vi "General_Slice 1D Array (U32).vi"(8 "Error":errorcluster, 9 "Slice":string caption="subset (i:j)", 11 "Array":u32[](array[colorbox])) -> (0 "Error Out":errorcluster, 3 "Array Out":u32[](array[colorbox]))   [LabVIEW 2009]
doc: "Modified OpenG vi Slice a 1D color array"
panel:
  # "Slice 1D Array.vi\n\nReturns a subset from array\n\nPlease visit http://www.OpenG.org to learn about the\nOpen Source LabVIEW software movement.\n\nNOTICE -- YOU MUST LEAVE THIS NOTICE IN PLACE.  PER THE TERMS OF THE LICENSE BELOW, YOU MAY SUBLICENSE THIS SOFTWARE \nIN ANY WAY THAT DOES NOT CONFLICT WITH THIS LICENSE.\n\n### BSD License (http://www.opensource.org/licenses/bsd-license.php) Begin ###\n \nCopyright (c) 2002, Jim Kring <jim@jimkring.com>\nCopyright (c) 2002, Cal-Bay Systems, Inc. <info@calbay.com>\n\nAll rights reserved.\n\nRedistribution and use in source and binary forms, with or without modification, are permitted provided that the following conditions are met:\n\n    * Redistributions of source code must retain the above copyright notice, this list of conditions and the following disclaimer.\n    * Redistributions in binary form must reproduce the above copyright notice, this list of conditions and the following disclaimer in the \n       documentation and/or other materials provided with the distribution.\n    * Neither the name of SciWare, James Kring, Inc., nor the names of its contributors may be used to endorse or promote products derived \n       from this software without specific prior written permission.\n\nTHIS SOFTWARE IS PROVIDED BY THE COPYRIGHT HOLDERS AND CONTRIBUTORS \"AS IS\" AND ANY EXPRESS OR IMPLIED WARRANTIES, \nINCLUDING, BUT NOT LIMITED TO, THE IMPLIED WARRANTIES OF MERCHANTABILITY AND FITNESS FOR A PARTICULAR PURPOSE ARE \nDISCLAIMED. IN NO EVENT SHALL THE COPYRIGHT OWNER OR CONTRIBUTORS BE LIABLE FOR ANY DIRECT, INDIRECT, INCIDENTAL,\n SPECIAL, EXEMPLARY, OR CONSEQUENTIAL DAMAGES (INCLUDING, BUT NOT LIMITED TO, PROCUREMENT OF SUBSTITUTE GOODS OR \nSERVICES; LOSS OF USE, DATA, OR PROFITS; OR BUSINESS INTERRUPTION) HOWEVER CAUSED AND ON ANY THEORY OF LIABILITY, \nWHETHER IN CONTRACT, STRICT LIABILITY, OR TORT (INCLUDING NEGLIGENCE OR OTHERWISE) ARISING IN ANY WAY OUT OF THE USE \nOF THIS SOFTWARE, EVEN IF ADVISED OF THE POSSIBILITY OF SUCH DAMAGE.\n\n### BSD License End ###"
  # "[OpenG VI Tags] ***Do Not Remove***\nSVN Revision = 593\nSVN Revision Date = 2007-01-18 16:52:28 -0800 (Thu, 18 Jan 2007)\nPackage = oglib_array-2.7-1\nDepends = oglib_string-2.6-1"
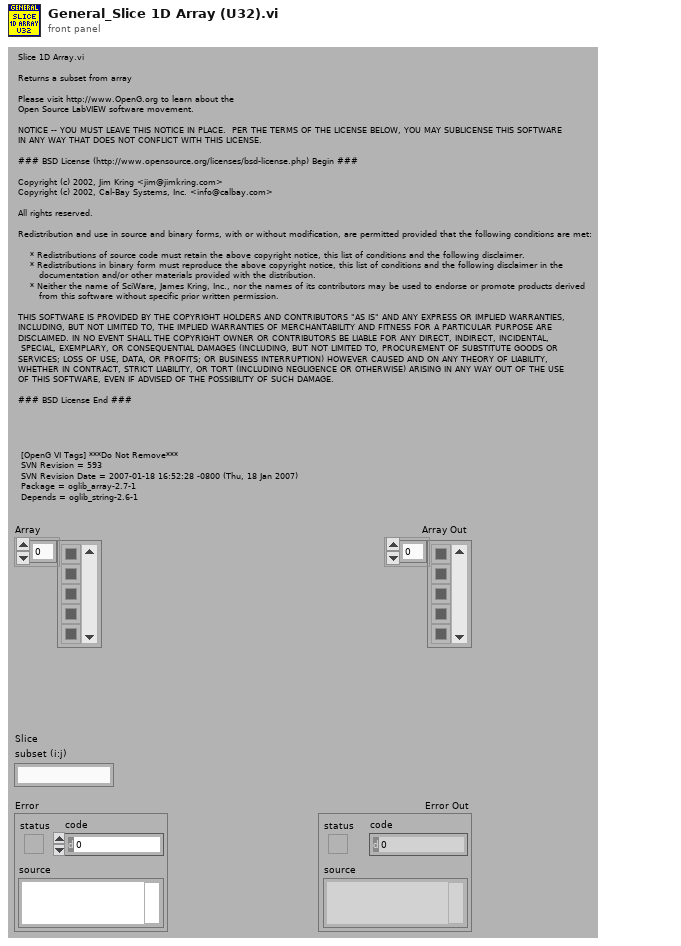
[diagram p1: front panel]
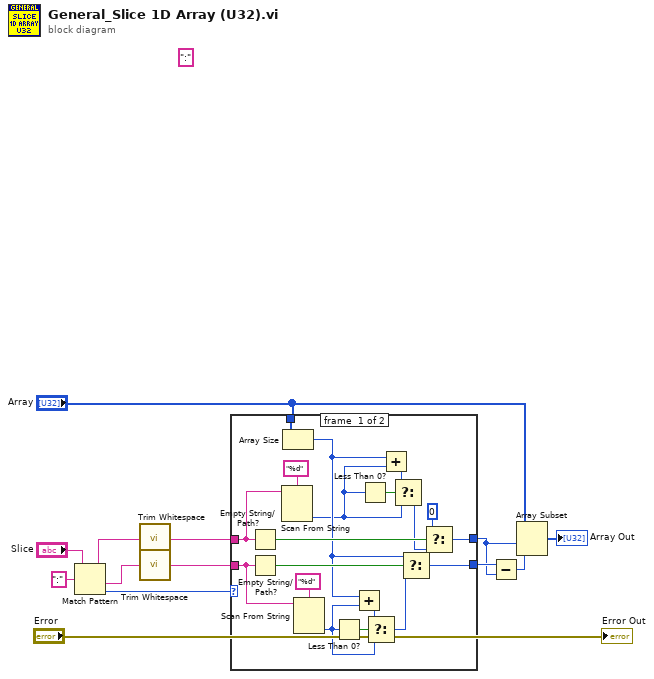
[diagram p0: block diagram]
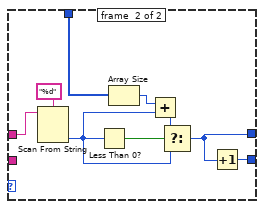
[diagram p2: hidden frame]
diagram:
  (unwired) ":"
  n1 = Match Pattern(string="Slice", regular expression=":" ("search string/char (-)")) -> (before substring=w7:string, after substring=w5:string, offset past match=w8:i32)  [unwired: 1 in, 1 out]
  n2 = call <vilib>:"Trim Whitespace.vi"("string"=w7) -> ("trimmed string"=w6:string)  [unwired: 1 in]
  n3 = call <vilib>:"Trim Whitespace.vi"("string"=w5) -> ("trimmed string"=w4:string)  [unwired: 1 in]
  n4 = case shown="-1" w8 {
    tunnel: [w23 w34] -> w13
    tunnel: [w24 w33] -> w12
    tunnel: "Array" -> [w29 w39]
    tunnel: w6 -> [w26 w40]
    tunnel: w4 -> [w30 _]
    frame #0 {
      n5 = Empty String/Path?(string/path=w26) -> (empty?=w28:bool)
      n6 = Empty String/Path?(string/path=w30) -> (empty?=w32:bool)
      n7 = Scan From String(format string="%d" ("Format String"), input string=w26) -> (output 1=w15:i32)  [unwired: 3 in, 3 out]
      n8 = Array Size(array=w29) -> (size(s)=w17:i32)
      n9 = Scan From String(format string="%d" ("Format String"), input string=w30) -> (output 1=w20:i32)  [unwired: 3 in, 3 out]
      n10 = Less Than 0?(x=w20) -> (x < 0?=w22:bool)
      n11 = Add(x=w17, y=w20) -> (x+y=w21:i32)
      n12 = Less Than 0?(x=w15) -> (x < 0?=w18:bool)
      n13 = Select(t=w21, s=w22, f=w20) -> (s? t:f=w19:i32)
      n14 = Add(x=w17, y=w15) -> (x+y=w16:i32)
      n15 = Select(t=w16, s=w18, f=w15) -> (s? t:f=w14:i32)
      n16 = Select(t=w17, s=w32, f=w19) -> (s? t:f=w23:i32)
      n17 = Select(t=0 ("length"), s=w28, f=w14) -> (s? t:f=w24:i32)
    }
    frame #1 {
      n18 = Scan From String(format string="%d" ("Format String"), input string=w40) -> (output 1=w35:i32)  [unwired: 3 in, 3 out]
      n19 = Less Than 0?(x=w35) -> (x < 0?=w38:bool)
      n20 = Array Size(array=w39) -> (size(s)=w37:i32)
      n21 = Add(x=w37, y=w35) -> (x+y=w36:i32)
      n22 = Select(t=w36, s=w38, f=w35) -> (s? t:f=w33:i32)
      n23 = Increment(x=w33) -> (x+1=w34:i32)
    }
  }
  n24 = Subtract(x=w13, y=w12) -> (x-y=w3:i32)
  n25 = Array Subset(array="Array", index=w12, length=w3) -> (→"Array Out":u32[])
  "Error Out" <- "Error"
